vi "Build Report String.vi"(8 "error in (no error)":errorcluster, 10 "Report Data":T1, 11 "Mouse Macro in":refnum<class "Mouse Macro.lvclass">) -> (0 "error out":errorcluster, 2 "Report String":string, 3 "Mouse Macro out":refnum<class "Mouse Macro.lvclass">)   [LabVIEW 2020, in "MacroAssert.lvlib" / "Mouse Macro.lvclass"]
doc: "Builds a string using <B>Step</B> and <B>Report Data</B> to be included in a report."
uses:
  Mouse Macro.lvclass
  Mouse Macro.lvclass/Mouse Macro.ctl
  Macro Step/Macro Step.lvclass
  CTLs/Report Data.ctl
  MacroAssert.lvlib
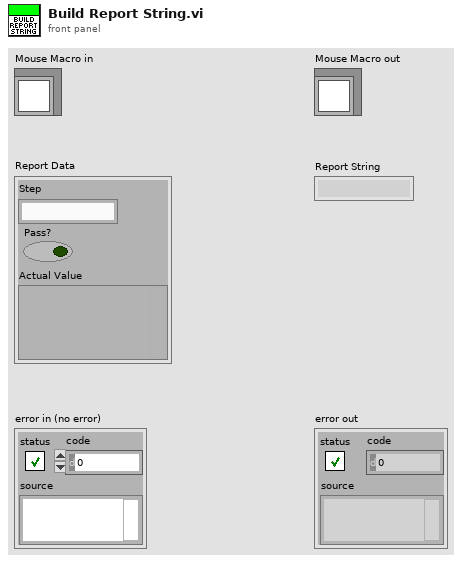
[diagram p1: front panel]
types:
  T1 = typedef "MacroAssert.lvlib/Report Data.ctl" = cluster{"Step":string, "Pass?":bool, "Actual Value":variant}
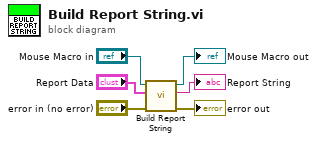
[diagram p0: block diagram]
diagram:
  n1 = call-parent "Build Report String.vi"("error in (no error)"="error in (no error)", "Report Data"="Report Data", "Step in"="Mouse Macro in") -> ("error out"=→"error out":errorcluster, "Report String"=→"Report String":string, "Step out"=→"Mouse Macro out":refnum<class "Mouse Macro.lvclass">)  [unwired: 6 in]
